vi "ENPH 354 Assignment 2 - Q2.vi"() -> ()   [LabVIEW 2021]
panel:
  out "XY Graph":cluster{i32[], dbl[]}(graph)
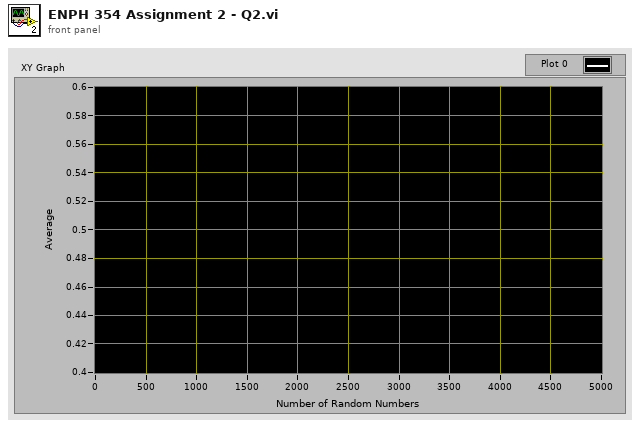
[diagram p1: front panel]
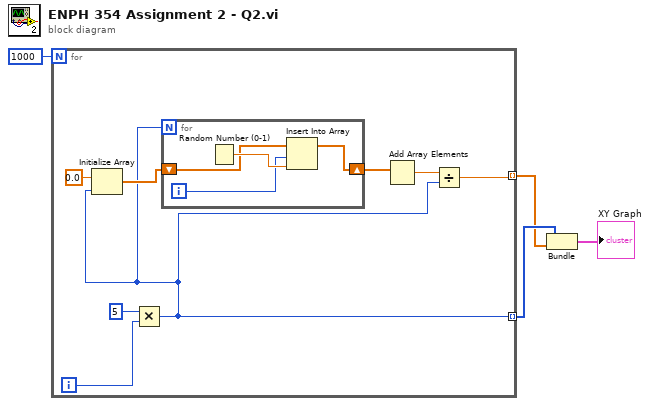
[diagram p0: block diagram]
diagram:
  n1 = for {
    N: 1000 -> [_]
    tunnel: [w7] -> w1 mode=indexing
    tunnel: [w5] -> w2 mode=indexing
    i -> [w6]
    n2 = Multiply(x=5, y=w6) -> (x*y=w5:i32)
    n3 = Initialize Array(0.0 ("element"), w5) -> (w10:dbl[])
    n4 = for {
      N: w5 -> [_]
      shift-right: [w13] -> w9
      shift-left: w10 -> [w15]
      i -> [w14]
      n5 = Random Number (0-1)() -> (number: 0 to 1=w16:dbl)
      n6 = Insert Into Array(array=w15, index=w14, new element=w16) -> (w13:dbl[])
    }
    n7 = Add Array Elements(numeric array=w9) -> (sum=w8:dbl)
    n8 = Divide(x=w8, y=w5) -> (x/y=w7:dbl)
  }
  n9 = Bundle(w2, w1) -> (→"XY Graph":cluster{i32[], dbl[]})  [unwired: 1 in]
